vi "svx_DAQ_FindChannelChanges.vi"(9 "New Value":T1[](array[typedef]) {"Max" min=0.0 format="± %^#_4g"; "Channel Type" items=["Voltage (V)"=0, "Charge (C)"=9, "-"=99, "SPL (Pa)"=3, "Force (lbf)"=6, "Force (N)"=1, "Acceleration (g) - IEPE"=2, "Acceleration (g) - Charge"=12, "Acceleration (g) - 4 wire DC Voltage"=22, "Velocity (in/s)"=7, "Velocity (mm/s)"=8, "Prox Probe (mil)"=4, "Prox Probe (mm)"=5]}, 11 "Old Value":T1[](array[typedef]) {"Max" min=0.0 format="± %^#_4g"; "Channel Type" items=["Voltage (V)"=0, "Charge (C)"=9, "-"=99, "SPL (Pa)"=3, "Force (lbf)"=6, "Force (N)"=1, "Acceleration (g) - IEPE"=2, "Acceleration (g) - Charge"=12, "Acceleration (g) - 4 wire DC Voltage"=22, "Velocity (in/s)"=7, "Velocity (mm/s)"=8, "Prox Probe (mil)"=4, "Prox Probe (mm)"=5]}) -> (1 "Channel Array Out":T1[](array[typedef]) {"Max" min=0.0 format="± %^#_4g"; "Channel Type" items=["Voltage (V)"=0, "Charge (C)"=9, "-"=99, "SPL (Pa)"=3, "Force (lbf)"=6, "Force (N)"=1, "Acceleration (g) - IEPE"=2, "Acceleration (g) - Charge"=12, "Acceleration (g) - 4 wire DC Voltage"=22, "Velocity (in/s)"=7, "Velocity (mm/s)"=8, "Prox Probe (mil)"=4, "Prox Probe (mm)"=5]})   [LabVIEW 2017, in "SVX NI-DAQmx AI Configuration XControl.xctl"]
uses:
  <vilib>/addons/Sound and Vibration/svt_DAQmx/Configuration XControl/SVX NI-DAQmx AI Configuration XControl.xctl
  <vilib>/addons/Sound and Vibration/svt_DAQmx/Configuration XControl/Controls/svx_DAQ_ChannelInfo.ctl
  <vilib>/addons/Sound and Vibration/svt_DAQmx/Configuration XControl/Controls/svx_DAQ_ChannelType.ctl
  <vilib>/addons/Sound and Vibration/svt_DAQmx/Configuration XControl/Controls/svx_DAQ_Coupling.ctl
  <vilib>/addons/Sound and Vibration/svt_DAQmx/Configuration XControl/Controls/svx_DAQ_Excitation.ctl
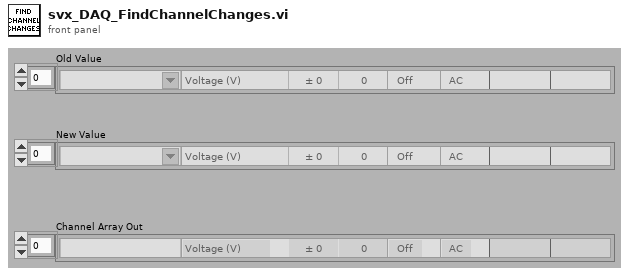
[diagram p1: front panel]
types:
  T1 = typedef "SVX NI-DAQmx AI Configuration XControl.xctl/svx_DAQ_ChannelInfo.ctl" = cluster{"Initialized?":bool, "DAQmx Channel":tag, "Channel Type":T2, "Max":dbl, "Sensitivity":dbl, "Excitation":bool, "Coupling":T3, "Location":string, "Orientation":string, "excitation":T4}
  T2 = typedef "SVX NI-DAQmx AI Configuration XControl.xctl/svx_DAQ_ChannelType.ctl" = u16
  T3 = typedef "SVX NI-DAQmx AI Configuration XControl.xctl/svx_DAQ_Coupling.ctl" = enum16{"AC", "DC"}
  T4 = typedef "svx_DAQ_Excitation.ctl" = enum16{"Off", "Min", "Max"}
  T5 = cluster{"Initialized?":bool, "DAQmx Channel":bool, "Channel Type":bool, "Max":bool, "Sensitivity":bool, "Excitation":bool, "Coupling":bool, "Location":bool, "Orientation":bool, "excitation":bool}[]
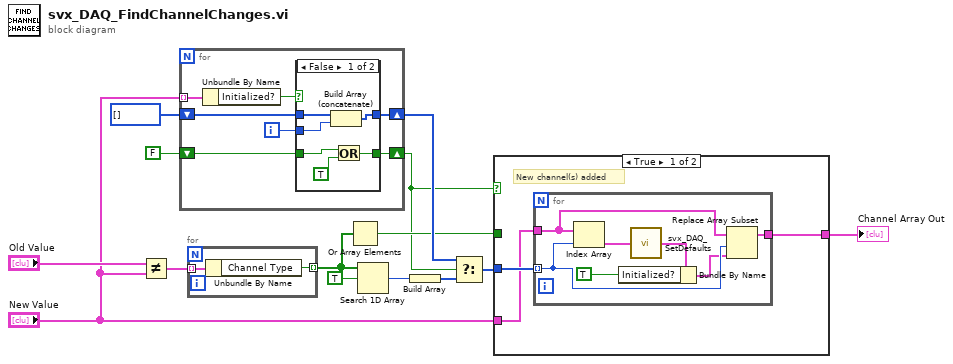
[diagram p0: block diagram]
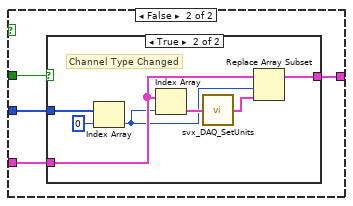
[diagram p2: hidden frame]
diagram:
  n1 = Not Equal?(x="Old Value", y="New Value") -> (x != y?=w14:T5)
  n2 = for {
    tunnel: "New Value" -> [w15] mode=indexing
    shift-right: [w20] -> w11
    shift-left: i32[] [] -> [w19]
    shift-right: [w17] -> w4
    shift-left: FALSE -> [w16]
    i -> [w18]
    n3 = Unbundle By Name(w15) -> ("Initialized?"=w21:bool)
    n4 = case shown="False" w21 {
      tunnel: [w27 w29] -> w20
      tunnel: w19 -> [w25 w29]
      tunnel: w18 -> [w26 _]
      tunnel: [w23 w28] -> w17
      tunnel: w16 -> [w22 w28]
      frame False {
        n5 = Build Array (concatenate)(w25, w26) -> (w27:i32[])
        n6 = Or(x=w22, y=TRUE) -> (x .or. y?=w23:bool)
      }
      frame True {
      }
    }
  }
  n7 = for {
    tunnel: w14 -> [w31] mode=indexing
    tunnel: [w30] -> w12 mode=indexing
    n8 = Unbundle By Name(w31) -> ("Channel Type"=w30:bool)
  }
  n9 = Or Array Elements(Boolean array=w12) -> (logical OR=w6:bool)
  n10 = Search 1D Array(1D array=w12, element=TRUE) -> (index of element=w10:i32)  [unwired: 1 in]
  n11 = Build Array(w10) -> (w9:i32[])
  n12 = Select(t=w11, s=w4, f=w9) -> (s? t:f=w7:i32[])
  n13 = case shown="True" w4 {
    tunnel: "New Value" -> [w33 w42]
    tunnel: w7 -> [w34 w44]
    tunnel: [w32 w43] -> w1
    tunnel: w6 -> [_ w45]
    frame True {
      # "New channel(s) added"
      n14 = for {
        tunnel: w34 -> [w41] mode=indexing
        tunnel: w33 -> [w40]
        tunnel: [w39] -> w32
        n15 = Index Array(array=w40, index=w41) -> (element=w37:T1)
        n16 = call <vilib>:"svx_DAQ_SetDefaults.vi"("Channel Information In"=w37) -> ("Channel Information Out"=w36:T1)  [unwired: 14 in]
        n17 = Bundle By Name(cluster=w36, "Initialized?"=TRUE) -> (w35:T1)
        n18 = Replace Array Subset(array=w40, new element=w35, index=w41) -> (w39:T1[])
      }
    }
    frame False {
      n19 = case shown="True" w45 {
        tunnel: w42 -> [w46 w52]
        tunnel: w44 -> [_ w49]
        tunnel: [w46 w50] -> w43
        frame False {
        }
        frame True {
          # "Channel Type Changed"
          n20 = Index Array(array=w49, index=0) -> (element=w48:i32)
          n21 = Index Array(array=w52, index=w48) -> (element=w53:T1)
          n22 = call <vilib>:"svx_DAQ_SetUnits.vi"("Channel Information In"=w53) -> ("Channel Information Out"=w51:T1)  [unwired: 4 in]
          n23 = Replace Array Subset(array=w52, new element=w51, index=w48) -> (w50:T1[])
        }
      }
    }
  }
  "Channel Array Out" <- w1
